vi "List.vi"(4 "error in (no error)":errorcluster) -> (0 "error out":errorcluster, 1 "Serial numbers":i32[](array[numeric]), 2 "Device id strings":string[](array[string]))   [LabVIEW 2014, in "MBUG-2820.lvlib"]
doc: "Create a list of available MBUG-2820 devices. The list is provided as array of device id strings and as array of device serial numbers. Elements of either arrays can be passed directly to the Open function to open the respective device."
uses:
  <instrlib>/MBUG-2820/MBUG-2820.lvlib
  <instrlib>/MBUG-2820/mbugdll.dll
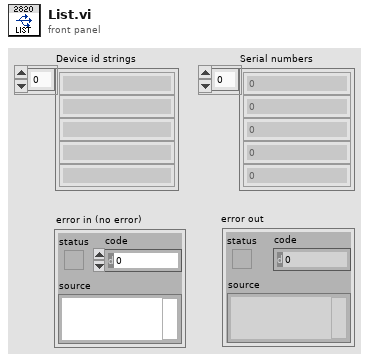
[diagram p1: front panel]
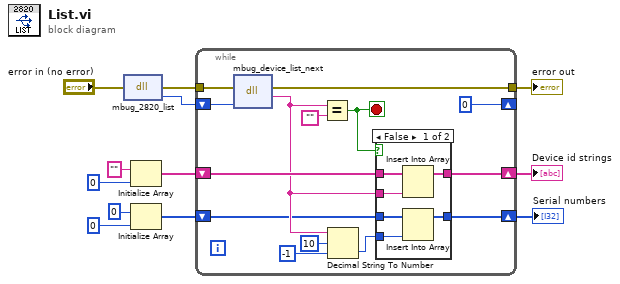
[diagram p0: block diagram]
diagram:
  n1 = dll-call lib="C:/Programme/National Instruments/LabVIEW 2014/instr.lib/MBUG-2820/mbugdll.dll" fn="mbug_2820_list"(error in="error in (no error)") -> (error out=w12:errorcluster, "return type"=w11:i64)  [unwired: 2 in, 1 out]
  n2 = Initialize Array("", 0 ("dimension size")) -> (w7:string[])
  n3 = Initialize Array(0 ("dimension size"), 0 ("dimension size")) -> (w2:i32[])
  n4 = while {
    tunnel: w12 -> [w26]
    shift-right: [i64 0 ("return type")] -> _
    shift-left: w11 -> [w25]
    tunnel: [w23] -> w10
    shift-right: [w21] -> w8
    shift-left: w7 -> [w22]
    shift-right: [w14] -> w1
    shift-left: w2 -> [w13]
    stop <- w19 stop-if-true
    n5 = dll-call lib="C:/Programme/National Instruments/LabVIEW 2014/instr.lib/MBUG-2820/mbugdll.dll" fn="mbug_device_list_next"(error in=w26, "dev_list"=w25) -> (error out=w23:errorcluster, "return type"=w16:string)  [unwired: 3 in, 1 out]
    n6 = Equal?(x=w16, y="") -> (x = y?=w19:bool)
    n7 = Decimal String To Number(string=w16, offset=10, default (0L)=-1 ("default (0 I32)")) -> (number=w15:i32)  [unwired: 1 out]
    n8 = case shown="False" w19 {
      tunnel: w22 -> [w32 w34]
      tunnel: w16 -> [w30 _]
      tunnel: [w31 w34] -> w21
      tunnel: w15 -> [w29 _]
      tunnel: [w28 w33] -> w14
      tunnel: w13 -> [w27 w33]
      frame False {
        n9 = Insert Into Array(array=w32, new element=w30) -> (w31:string[])  [unwired: 1 in]
        n10 = Insert Into Array(array=w27, new element=w29) -> (w28:i32[])  [unwired: 1 in]
      }
      frame True {
      }
    }
  }
  "error out" <- w10
  "Device id strings" <- w8
  "Serial numbers" <- w1
